vi "Emballage check lot terminé.vi"(0 "N° carton en cours":i32=7, 1 "Nb valves dans carton":i32=7, 2 "Nombre de pièce emballées":i16, 7 "date de prod de la piece en cours":string, 11 "Tab n° carton - nb ds carton":i32[][](array[numeric]), 12 "Tableau lots OUT":string[][](array[string])=[["0810", "13"], ["0811", "7"], ["0812", "31"]]) -> (3 "Changer de carton":bool=TRUE, 8 "Affiche \"scan lot suivant\"":bool=TRUE, 14 "indice lot suivant":i32=2)   [LabVIEW 2020]
panel:
  out "Pas bon lot?":bool
  out "qtté  du lot":i32=7
  # "0926"
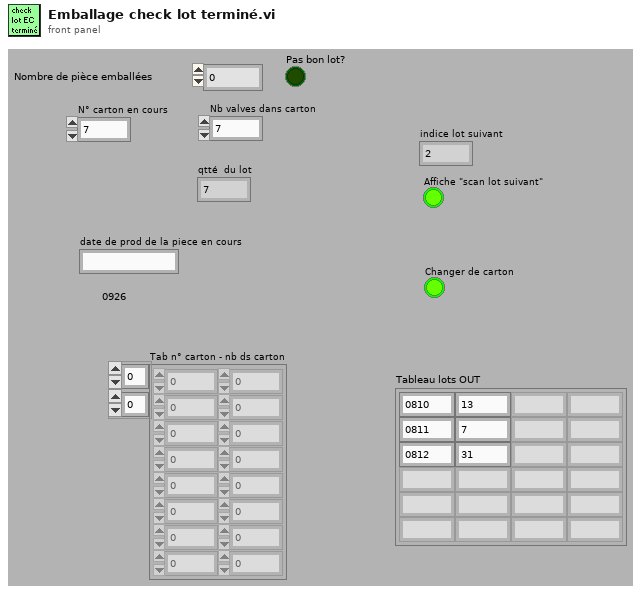
[diagram p1: front panel]
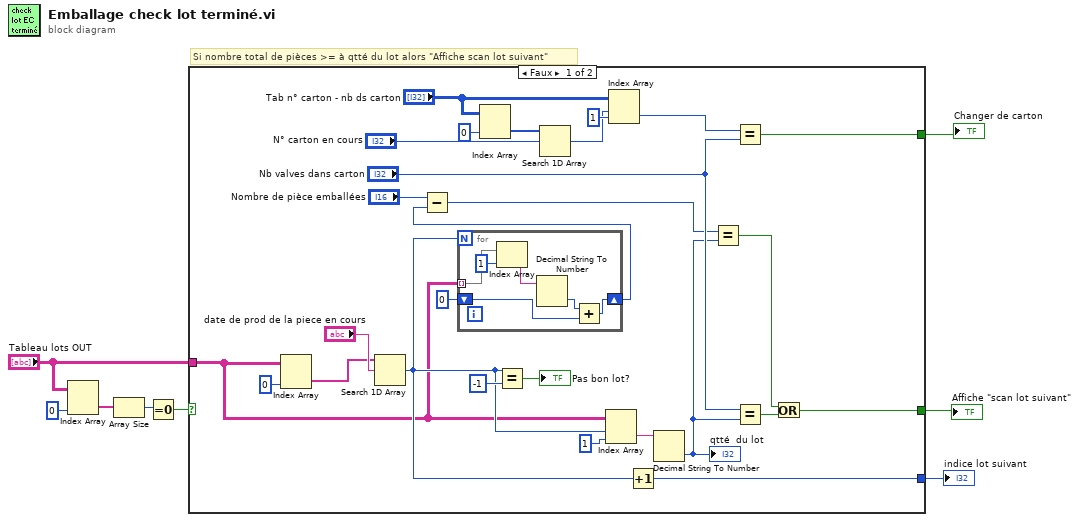
[diagram p0: block diagram]
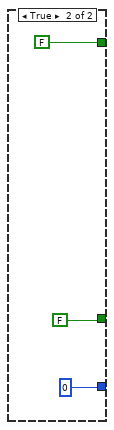
[diagram p2: hidden frame]
diagram:
  # "Si nombre total de pièces >= à qtté du lot alors \"Affiche scan lot suivant\""
  n1 = Index Array(array="Tableau lots OUT", index (col)=0 ("indice désactivé (col)")) -> (element=w4:string[])  [unwired: 1 in]
  n2 = Array Size(array=w4) -> (size(s)=w3:i32)
  n3 = Equal To 0?(x=w3) -> (x = 0?=w2:bool)
  n4 = case shown="Faux" w2 {
    tunnel: "Tableau lots OUT" -> [w12 _]
    tunnel: [w23 FALSE] -> w8
    tunnel: [w31 0] -> w7
    tunnel: [w22 FALSE] -> w1
    frame False {
      n5 = Index Array(array=w12, index (col)=0 ("indice désactivé (col)")) -> (element=w14:string[])  [unwired: 1 in]
      n6 = Search 1D Array(1D array=w14, element="date de prod de la piece en cours") -> (index of element=w13:i32)  [unwired: 1 in]
      n7 = for {
        N: w13 -> [_]
        tunnel: w12 -> [w40] mode=indexing
        shift-right: [w38] -> w10
        shift-left: 0 -> [w36]
        n8 = Index Array(array=w40, index=1 ("indice")) -> (element=w39:string)
        n9 = Decimal String To Number(string=w39) -> (number=w37:i32)  [unwired: 2 in, 1 out]
        n10 = Add(x=w37, y=w36) -> (x+y=w38:i32)
      }
      n11 = Subtract(x="Nombre de pièce emballées", y=w10) -> (x-y=w9:i32)
      n12 = Index Array(array="Tab n° carton - nb ds carton", index (col)=0 ("indice désactivé (col)")) -> (element=w29:i32[])  [unwired: 1 in]
      n13 = Equal?(x=w13, y=-1) -> (x = y?=→"Pas bon lot?":bool)
      n14 = Search 1D Array(1D array=w29, element="N° carton en cours") -> (index of element=w26:i32)  [unwired: 1 in]
      n15 = Index Array(array=w12, index (row)=w13, index (col)=1 ("indice désactivé (col)")) -> (element=w32:string)
      n16 = Index Array(array="Tab n° carton - nb ds carton", index (row)=w26, index (col)=1 ("indice désactivé (col)")) -> (element=w24:i32)
      n17 = Increment(x=w13) -> (x+1=w31:i32)
      n18 = Decimal String To Number(string=w32) -> (number=w17:i32)  [unwired: 2 in, 1 out]
      "qtté  du lot" <- w17
      n19 = Equal?(x=w9, y=w17) -> (x = y?=w16:bool)
      n20 = Equal?(x=w24, y="Nb valves dans carton") -> (x = y?=w22:bool)
      n21 = Equal?(x="Nb valves dans carton", y=w17) -> (x = y?=w25:bool)
      n22 = Or(x=w16, y=w25) -> (x .or. y?=w23:bool)
    }
    frame True {
    }
  }
  "Affiche \"scan lot suivant\"" <- w8
  "indice lot suivant" <- w7
  "Changer de carton" <- w1
